vi "GetSensor.vi"(5 "DB Serial No. IN":string) -> (0 "Manufacturer":string, 1 "Batch No.":string, 2 "Wafer No.":string, 3 "Record found?":bool, 4 "Device Category:":string(combo)="ATLAS18SS")   [LabVIEW 2018]
uses:
  globals/QC_RunInformation.vi
panel:
  out "error out":errorcluster
  out "Lookup file":string
  out "line found":string
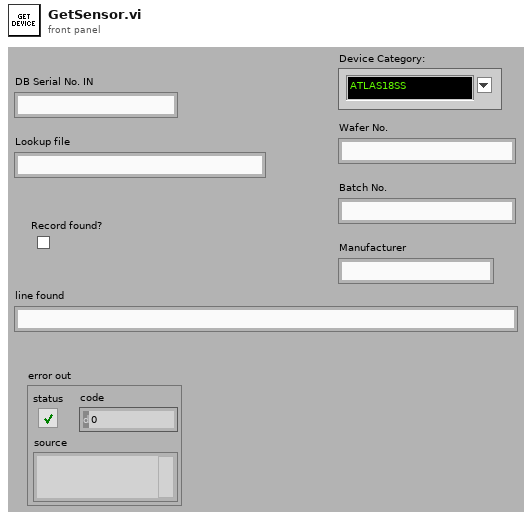
[diagram p1: front panel]
types:
  T1 = cluster{"Institute":string, "Manufacturers":string[], "Devices":string[], "Serialnumbers Lookup DB":string, "Data directory":string, "Backup & screenshot directory":string, "List of known users":string[], "Measurement switch not used":bool, "Measurement Switch":string, "DUT Switch":string, "Rseries IV [MOhm]":string, "Rshunt IV [MOhm]":string, "Rseries CV [MOhm]":string, "DC blocking Cap [µF]":string, "Rseries LCR [MOhm]":string, "Rseries stability [MOhm]":string, "Rshunt stability [MOhm]":string, "Rseries striptest bias [MOhm]":string, "Rseries strip pinhole [MOhm]":string}
  T2 = cluster{"Sensor Serial No.:":string, "Wafer:":string, "Batch:":string, "Manufacturer:":string, "Device Category:":string, "Database Serial No.:":string, "Institution":string, "Current Location":string, "Assembled?":bool, "Component:":string}
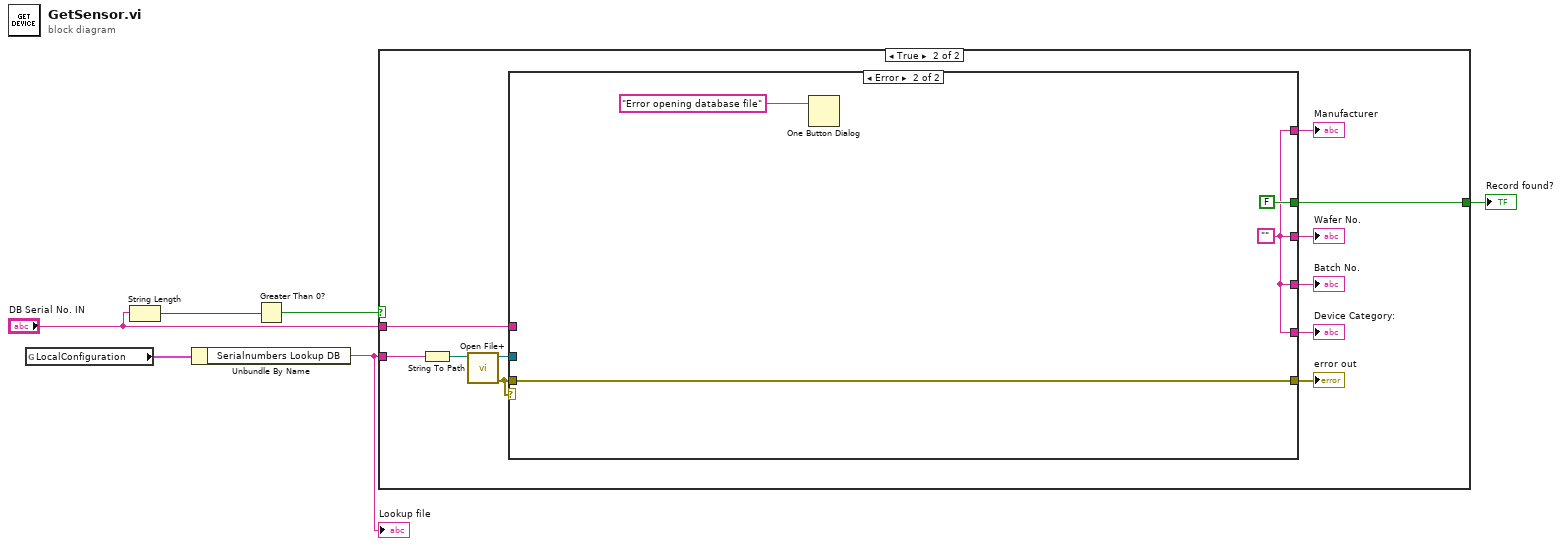
[diagram p0: block diagram]
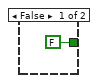
[diagram p2: hidden frame]
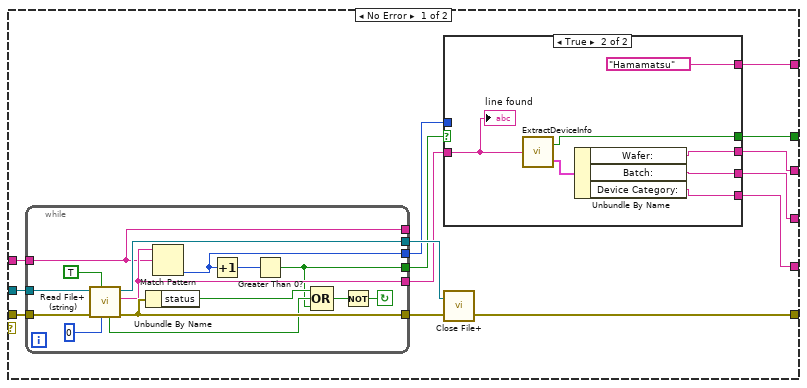
[diagram p3: hidden frame]
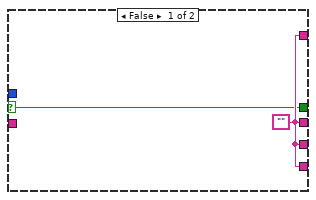
[diagram p4: hidden frame]
diagram:
  n1 = global read "QC_RunInformation.vi" "LocalConfiguration"() -> (w2:T1)
  n2 = String Length(string="DB Serial No. IN") -> (length=w4:i32)
  n3 = Unbundle By Name(w2) -> ("Serialnumbers Lookup DB"=w1:string)
  "Lookup file" <- w1
  n4 = Greater Than 0?(x=w4) -> (x > 0?=w3:bool)
  n5 = case shown="True" w3 {
    tunnel: w1 -> [_ w16]
    tunnel: "DB Serial No. IN" -> [_ w15]
    tunnel: [FALSE w14] -> w6
    frame False {
    }
    frame True {
      n6 = String To Path(string=w16) -> (path=w17:path)
      n7 = call <vilib>:"Open File+.vi"("file path (\" \")"=w17) -> ("error out"=w8:errorcluster, "refnum"=w18:refnum<file>)  [unwired: 7 in, 2 out]
      n8 = case shown="Error" w8 {
        tunnel: w18 -> [w32 _]
        tunnel: w15 -> [w29 _]
        tunnel: [w19 FALSE] -> w14
        tunnel: w8 -> [w28 w58]
        tunnel: [w27 w58] -> w11
        tunnel: [w23 w57] -> w13
        tunnel: [w22 w57] -> w12
        tunnel: [w21 w57] -> w10
        tunnel: [w20 w57] -> w9
        frame No Error {
          n9 = while {
            tunnel: [w33] -> _
            tunnel: [w35] -> w24
            tunnel: [w36] -> w25
            tunnel: [w34] -> w26
            tunnel: w29 -> [w33]
            tunnel: [w42] -> w30
            tunnel: w28 -> [w43]
            tunnel: [w44] -> w31
            tunnel: w32 -> [w46]
            stop <- w37 continue-if-true
            n10 = call <vilib>:"Read File+ (string).vi"("count"=0, "line mode (characters:F)"=TRUE, "error in (no error)"=w43, "refnum"=w46) -> ("error out"=w42:errorcluster, "string"=w36:string, "dup refnum"=w44:refnum<file>, "EOF?"=w39:bool)  [unwired: 3 in, 1 out]
            n11 = Unbundle By Name(w42) -> ("status"=w40:bool)
            n12 = Match Pattern(string=w36, regular expression=w33) -> (offset past match=w35:i32)  [unwired: 1 in, 3 out]
            n13 = Increment(x=w35) -> (x+1=w41:i32)
            n14 = Greater Than 0?(x=w41) -> (x > 0?=w34:bool)
            n15 = Compound Arithmetic op=OR(w40, w39, w34) -> (w38:bool)
            n16 = Not(x=w38) -> (.not. x?=w37:bool)
          }
          n17 = case shown="True" w26 {
            selector: w26 -> [w48 _]
            tunnel: w25 -> [_ w56]
            tunnel: w24 -> [_ _]
            tunnel: [w49 "Hamamatsu" ("Manufacturer:")] -> w23
            tunnel: [w49 w53] -> w22
            tunnel: [w49 w52] -> w21
            tunnel: [w49 w51] -> w20
            tunnel: [w48 w55] -> w19
            frame False {
              w49 = ""
            }
            frame True {
              n18 = call "ExtractDeviceInfo.vi"("Line IN"=w56) -> ("valid record?"=w55:bool, "Device Info"=w54:T2)
              n19 = Unbundle By Name(w54) -> ("Wafer:"=w53:string, "Batch:"=w52:string, "Device Category:"=w51:string)
              "line found" <- w56
            }
          }
          n20 = call <vilib>:"Close File+.vi"("error in (no error)"=w30, "refnum"=w31) -> ("error out"=w27:errorcluster)  [unwired: 3 in, 2 out]
        }
        frame Error {
          w57 = ""
          n21 = One Button Dialog(message="Error opening database file") -> ()  [unwired: 1 in, 1 out]
        }
      }
      "Wafer No." <- w12
      "Manufacturer" <- w13
      "error out" <- w11
      "Batch No." <- w10
      "Device Category:" <- w9
    }
  }
  "Record found?" <- w6
